vi "R3_Data Collection.vi"() -> ()   [LabVIEW 2016]
uses:
  R3 Reactor Status v1.ctl
  <vilib>/Platform/TimedLoop/XDataNode/timing_clust.ctl
  <vilib>/Platform/TimedLoop/XDataNode/nitl_modes.ctl
  <vilib>/Platform/TimedLoop/XDataNode/wakeup.ctl
  R3 Pump Manual Control.ctl
  R3 pH Manual Control.ctl
  <vilib>/Platform/TimedLoop/XDataNode/XDataNode.xnode
  <vilib>/Platform/TimedLoop/XDataNode/XDNodeRunTimeDep.lvlib
  <vilib>/ptbypt/NI_PtbyPt.lvlib
  R3Variables.lvlib
panel:
  out "Numeric":i32
  out "Reactor 3 Status 3":T1 {"pH" format="%#_3g"}
  out "pH and DO":T2(graph)
  # "Click to stop all while loops and turn off all pumps/valves."
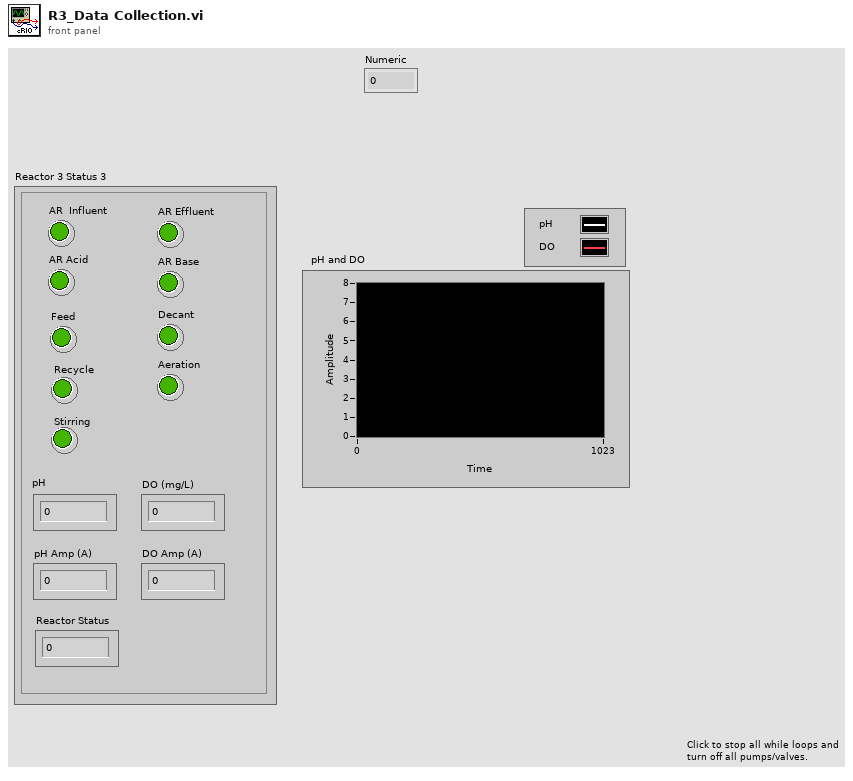
[diagram p1: front panel]
types:
  T1 = typedef "R3Variables.lvlib/R3 Reactor Status v1.ctl" = cluster{"AR  Influent":bool, "AR Effluent":bool, "AR Acid":bool, "AR Base":bool, "Feed":bool, "Aeration":bool, "Decant":bool, "pH":dbl, "DO (mg/L)":dbl, "pH Amp (A)":dbl, "DO Amp (A)":dbl, "Recycle":bool, "Stirring":bool, "Reactor Status":dbl}
  T2 = cluster{"[0]":dbl, "[1]":dbl, "[2]":dbl, "[3]":dbl, "[4]":dbl, "[5]":dbl, "[6]":dbl, "[7]":dbl, "[8]":dbl}
  T3 = typedef "R3Variables.lvlib/R3 Pump Manual Control.ctl" = cluster{"AR Influent":bool, "AR Effluent":bool, "PR Feed":bool, "PR Decant":bool, "PR Recycle":bool, "PR Aeration":bool, "Stirring":bool}
  T4 = typedef "R3Variables.lvlib/R3 pH Manual Control.ctl" = cluster{"Acid Pump":bool, "Base Pump":bool}
  T5 = typedef "XDNodeRunTimeDep.lvlib/timing_clust.ctl" = cluster{"Expected End [f-1]":u64, "Actual End [f-1]":u64, "Finished Late? [f-1]":bool, "Expected End [i-1]":u64, "Actual End [i-1]":u64, "Finished Late? [i-1]":bool, "Expected Start [i]":u64, "Actual Start [i]":u64, "Expected Start [f]":u64, "Actual Start [f]":u64, "Source Name":string, "Structure Name":string, "Period":i64, "Deadline":i64, "Offset":i64, "Start":i64, "Priority":i32, "Timeout":i32, "Mode":T6, "Wakeup Reason":T7, "Error":errorcluster, "Source Type":string, "Secondary Source Type":string, "Global End Time":u64, "Global Start Time":u64, "Frame Duration":u64, "Iteration Duration":u64, "Assigned CPU":i32, "I/O Scan Engine Mode":u32}
  T6 = typedef "XDNodeRunTimeDep.lvlib/nitl_modes.ctl" = enum32{"No Change", "Process missed periods, maintain original phase", "Discard missed periods, maintain original phase", "Process missed periods, ignore original phase", "Discard missed periods, ignore original phase"}
  T7 = typedef "XDNodeRunTimeDep.lvlib/wakeup.ctl" = enum32{"Normal", "Aborted", "Asynchronous wakeup", "Timing source error", "Timed loop error", "Timeout"}
  T8 = cluster{"Array of Double[0]":dbl, "Array of Double[1]":dbl, "Array of Double[2]":dbl, "Array of Double[3]":dbl, "Array of Double[4]":dbl, "Array of Double[5]":dbl, "Array of Double[6]":dbl, "Array of Double[7]":dbl, "Array of Double[8]":dbl}
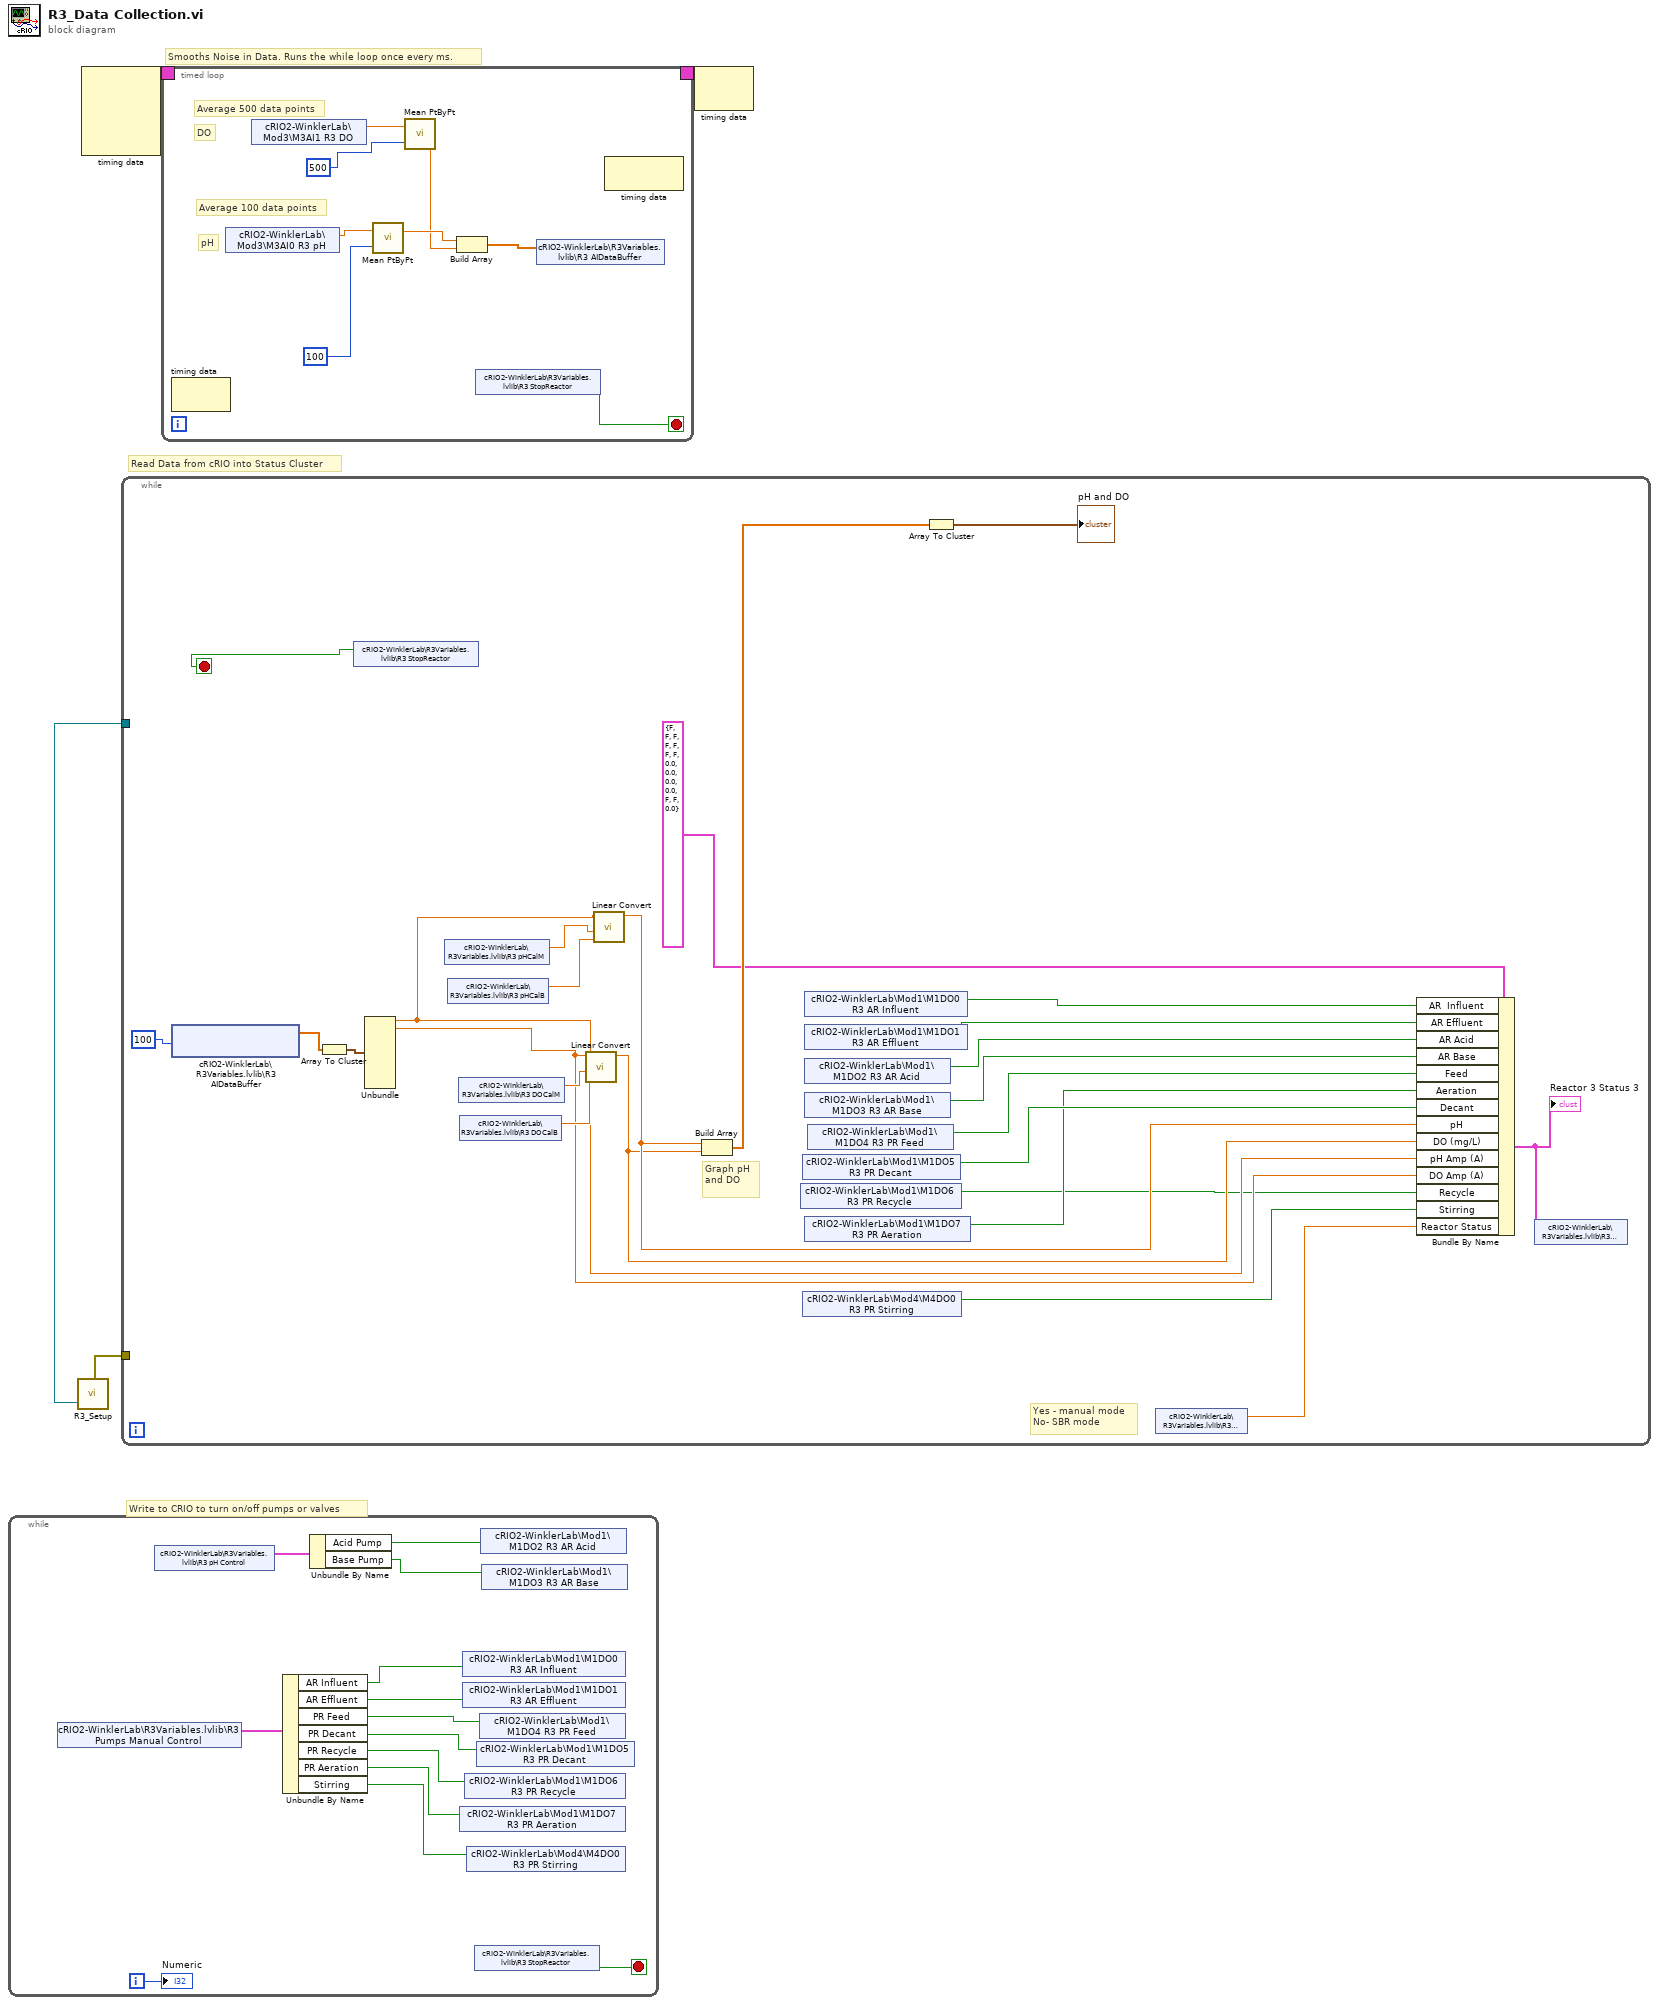
[diagram p0: block diagram]
diagram:
  # "Smooths Noise in Data. Runs the while loop once every ms."
  # "Write to CRIO to turn on/off pumps or valves"
  # "Read Data from cRIO into Status Cluster"
  n1 = while {
    i -> [w16]
    stop <- w15 stop-if-true
    n2 = shared-variable "cRIO2-WinklerLab\\R3Variables.lvlib\\R3 Pumps Manual Control"() -> (w14:T3)  [unwired: 1 in, 1 out]
    n3 = shared-variable "cRIO2-WinklerLab\\R3Variables.lvlib\\R3 pH Control"() -> (w17:T4)  [unwired: 1 in, 1 out]
    n4 = Unbundle By Name(w14) -> ("AR Influent"=w13:bool, "AR Effluent"=w12:bool, "PR Feed"=w11:bool, "PR Decant"=w5:bool, "PR Recycle"=w10:bool, "PR Aeration"=w9:bool, "Stirring"=w8:bool)
    n5 = Unbundle By Name(w17) -> ("Acid Pump"=w7:bool, "Base Pump"=w6:bool)
    n6 = shared-variable "cRIO2-WinklerLab\\Mod1\\M1DO7 R3 PR Aeration"(w9) -> ()  [unwired: 1 in, 1 out]
    n7 = shared-variable "cRIO2-WinklerLab\\Mod1\\M1DO0 R3 AR Influent"(w13) -> ()  [unwired: 1 in, 1 out]
    n8 = shared-variable "cRIO2-WinklerLab\\Mod1\\M1DO1 R3 AR Effluent"(w12) -> ()  [unwired: 1 in, 1 out]
    n9 = shared-variable "cRIO2-WinklerLab\\Mod1\\M1DO6 R3 PR Recycle"(w10) -> ()  [unwired: 1 in, 1 out]
    n10 = shared-variable "cRIO2-WinklerLab\\Mod4\\M4DO0 R3 PR Stirring"(w8) -> ()  [unwired: 1 in, 1 out]
    n11 = shared-variable "cRIO2-WinklerLab\\R3Variables.lvlib\\R3 StopReactor"() -> (w15:bool)  [unwired: 1 in, 1 out]
    n12 = shared-variable "cRIO2-WinklerLab\\Mod1\\M1DO5 R3 PR Decant"(w5) -> ()  [unwired: 1 in, 1 out]
    n13 = shared-variable "cRIO2-WinklerLab\\Mod1\\M1DO4 R3 PR Feed"(w11) -> ()  [unwired: 1 in, 1 out]
    n14 = shared-variable "cRIO2-WinklerLab\\Mod1\\M1DO2 R3 AR Acid"(w7) -> ()  [unwired: 1 in, 1 out]
    n15 = shared-variable "cRIO2-WinklerLab\\Mod1\\M1DO3 R3 AR Base"(w6) -> ()  [unwired: 1 in, 1 out]
    "Numeric" <- w16
  }
  n16 = call "R3_Setup.vi"() -> ("tdms file out"=w2:refnum<k34>, "error out"=w1:errorcluster)  [unwired: 10 in]
  n17 = node-c288() -> (w4:T5)  [unwired: 4 in]
  n18 = while {
    tunnel: w1 -> [_]
    tunnel: w2 -> [_]
    stop <- w40 stop-if-true
    # "Yes - manual mode\nNo- SBR mode"
    # "Graph pH and DO"
    n19 = shared-variable "cRIO2-WinklerLab\\R3Variables.lvlib\\R3 AIDataBuffer"(u32 100 ("milliseconds to wait")) -> (w38:dbl[])  [unwired: 1 in, 2 out]
    n20 = Array To Cluster(array=w38) -> (cluster=w43:T8)
    n21 = shared-variable "cRIO2-WinklerLab\\R3Variables.lvlib\\R3 StopReactor"() -> (w40:bool)  [unwired: 1 in, 1 out]
    n22 = Unbundle(w43) -> ("Array of Double[0]"=w27:dbl, "Array of Double[1]"=w28:dbl)  [unwired: 7 out]
    n23 = shared-variable "cRIO2-WinklerLab\\R3Variables.lvlib\\R3 pHCalM"() -> (w37:dbl)  [unwired: 1 in, 1 out]
    n24 = shared-variable "cRIO2-WinklerLab\\R3Variables.lvlib\\R3 pHCalB"() -> (w36:dbl)  [unwired: 1 in, 1 out]
    n25 = shared-variable "cRIO2-WinklerLab\\R3Variables.lvlib\\R3 DOCalM"() -> (w35:dbl)  [unwired: 1 in, 1 out]
    n26 = shared-variable "cRIO2-WinklerLab\\R3Variables.lvlib\\R3 DOCalB"() -> (w34:dbl)  [unwired: 1 in, 1 out]
    n27 = call "Linear Convert.vi"("Intercept"=w34, "Slope"=w35, "Signal"=w28) -> ("Result"=w26:dbl)  [unwired: 8 in]
    n28 = call "Linear Convert.vi"("Intercept"=w36, "Slope"=w37, "Signal"=w27) -> ("Result"=w29:dbl)  [unwired: 8 in]
    n29 = Build Array(w29, w26) -> (w42:dbl[])
    n30 = shared-variable "cRIO2-WinklerLab\\Mod1\\M1DO6 R3 PR Recycle"() -> (w21:bool)  [unwired: 1 in, 1 out]
    n31 = shared-variable "cRIO2-WinklerLab\\Mod1\\M1DO5 R3 PR Decant"() -> (w23:bool)  [unwired: 1 in, 1 out]
    n32 = shared-variable "cRIO2-WinklerLab\\Mod4\\M4DO0 R3 PR Stirring"() -> (w20:bool)  [unwired: 1 in, 1 out]
    n33 = shared-variable "cRIO2-WinklerLab\\Mod1\\M1DO0 R3 AR Influent"() -> (w31:bool)  [unwired: 1 in, 1 out]
    n34 = shared-variable "cRIO2-WinklerLab\\Mod1\\M1DO1 R3 AR Effluent"() -> (w30:bool)  [unwired: 1 in, 1 out]
    n35 = shared-variable "cRIO2-WinklerLab\\Mod1\\M1DO2 R3 AR Acid"() -> (w19:bool)  [unwired: 1 in, 1 out]
    n36 = shared-variable "cRIO2-WinklerLab\\Mod1\\M1DO3 R3 AR Base"() -> (w18:bool)  [unwired: 1 in, 1 out]
    n37 = shared-variable "cRIO2-WinklerLab\\Mod1\\M1DO7 R3 PR Aeration"() -> (w22:bool)  [unwired: 1 in, 1 out]
    n38 = shared-variable "cRIO2-WinklerLab\\Mod1\\M1DO4 R3 PR Feed"() -> (w24:bool)  [unwired: 1 in, 1 out]
    n39 = Array To Cluster(array=w42) -> (cluster=→"pH and DO":T2)
    n40 = shared-variable "cRIO2-WinklerLab\\R3Variables.lvlib\\R3 Phase"() -> (w25:dbl)  [unwired: 1 in, 1 out]
    n41 = Bundle By Name(cluster=T1 {"AR  Influent"=FALSE, "AR Effluent"=FALSE, "AR Acid"=FALSE, "AR Base"=FALSE, "Feed"=FALSE, "Aeration"=FALSE, "Decant"=FALSE, "pH"=0.0, "DO (mg/L)"=0.0, "pH Amp (A)"=0.0, "DO Amp (A)"=0.0, "Recycle"=FALSE, "Stirring"=FALSE, "Reactor Status"=0.0} ("R3 Reactor Status"), "AR  Influent"=w31, "AR Effluent"=w30, "AR Acid"=w19, "AR Base"=w18, "Feed"=w24, "Aeration"=w22, "Decant"=w23, "pH"=w29, "DO (mg/L)"=w26, "pH Amp (A)"=w27, "DO Amp (A)"=w28, "Recycle"=w21, "Stirring"=w20, "Reactor Status"=w25) -> (w32:T1)
    "Reactor 3 Status 3" <- w32
    n42 = shared-variable "cRIO2-WinklerLab\\R3Variables.lvlib\\R3 Status"(w32) -> ()  [unwired: 1 in, 1 out]
  }
  n43 = timed-loop {
    timing: w4 -> [_]
    timing-out: [_] -> w3
    stop <- w48 stop-if-true
    # "Average 100 data points"
    # "pH"
    # "DO"
    # "Average 500 data points"
    n44 = node-c288() -> ()  [unwired: 1 in, 1 out]
    n45 = shared-variable "cRIO2-WinklerLab\\Mod3\\M3AI0 R3 pH"() -> (w44:dbl)  [unwired: 1 in, 1 out]
    n46 = shared-variable "cRIO2-WinklerLab\\Mod3\\M3AI1 R3 DO"() -> (w46:dbl)  [unwired: 1 in, 1 out]
    n47 = call <vilib>:"Mean PtByPt.vi"("x"=w44, "sample length"=100) -> ("mean"=w51:dbl)  [unwired: 2 in, 1 out]
    n48 = call <vilib>:"Mean PtByPt.vi"("x"=w46, "sample length"=500) -> ("mean"=w50:dbl)  [unwired: 2 in, 1 out]
    n49 = Build Array(w51, w50) -> (w47:dbl[])
    n50 = shared-variable "cRIO2-WinklerLab\\R3Variables.lvlib\\R3 StopReactor"() -> (w48:bool)  [unwired: 1 in, 1 out]
    n51 = shared-variable "cRIO2-WinklerLab\\R3Variables.lvlib\\R3 AIDataBuffer"(w47) -> ()  [unwired: 1 in, 1 out]
    n52 = node-c288() -> ()  [unwired: 1 in, 1 out]
  }
  n53 = node-c288(w3) -> ()  [unwired: 1 out]
